vi "Instructor Log.vi"() -> ()   [LabVIEW 2017]
uses:
  <vilib>/OPCUA/controls/Write Status.ctl
  <vilib>/OPCUA/controls/NodeId.ctl
  <vilib>/OPCUA/client/Multiple Write String.vi
  <vilib>/OPCUA/NI OPC UA Client.lvlib
panel:
  out "Log Loop":i32
  out "Send Loop":i32
  out "Chat Window":string
  in  "Node Status":T1 items=["Good"=0, "Uncertain_InitialValue"=1083310080, "Uncertain_LastUsableValue"=1083179008, "Uncertain_SensorNotAccurate"=1083375616, "Uncertain_EngineeringUnitsExceeded"=1083441152, "Bad_NoCommunication"=2150694912, "Bad_NotReadable"=2151284736, "Bad_NotWritable"=2151350272, "Bad_OutOfRange"=2151415808, "Bad_WaitingForInitialData"=2150760448]
  in  "Time Stamp":timestamp
  in  "Enter Text":string
  in  "Node Status":T1 items=["Good"=0, "Uncertain_InitialValue"=1083310080, "Uncertain_LastUsableValue"=1083179008, "Uncertain_SensorNotAccurate"=1083375616, "Uncertain_EngineeringUnitsExceeded"=1083441152, "Bad_NoCommunication"=2150694912, "Bad_NotReadable"=2151284736, "Bad_NotWritable"=2151350272, "Bad_OutOfRange"=2151415808, "Bad_WaitingForInitialData"=2150760448]
  in  "Time Stamp":timestamp
  in  "Stop Chat":bool
  in  "Send":bool
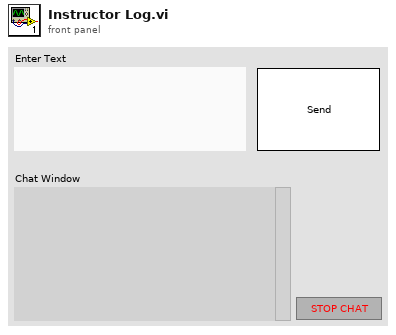
[diagram p1: front panel]
types:
  T1 = typedef "Write Status.ctl" = u32
  T2 = cluster{"message mode":enum16{"None", "Sign", "Sign and Encrypt"}, "security":enum16{"Basic256", "Basic128Rsa15"}}
  T3 = enum16{"open", "replace", "create", "open or create", "replace or create", "replace or create with confirmation"}
  T4 = typedef "OPC UA Client Refnum.ctl" = refnum<k21>
  T5 = typedef "NodeId.ctl" = string
  T6 = cluster{"node ID":T5, "value":string, "timestamp (current time)":timestamp, "node status":T1}
  T7 = cluster{"node ID":T5, "value":string, "timestamp (current time)":timestamp, "node status":T1}[]
  T8 = typedef "Subscription ID.ctl" = u32
  T9 = typedef "Subscription Data Change.ctl" = cluster{"node ID":T5, " value":variant, "timestamp":timestamp, "data type":T10, "status code":T11}
  T10 = typedef "Data Type.ctl" = u16
  T11 = typedef "OPC UA StatusCode.ctl" = u32
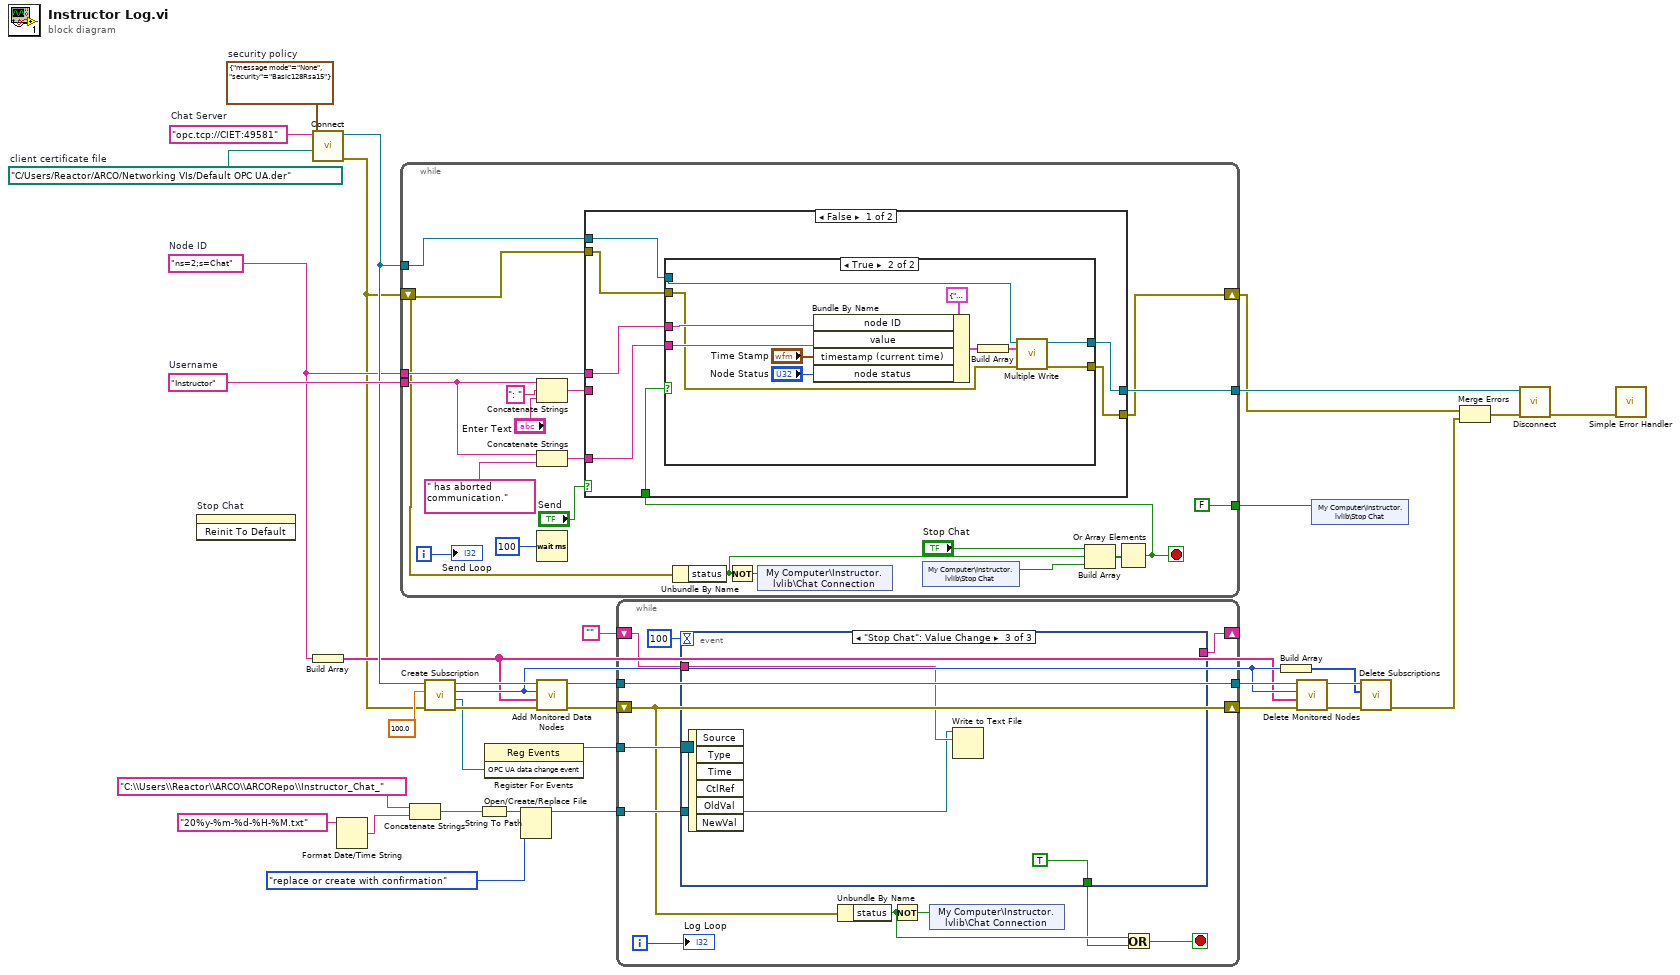
[diagram p0: block diagram]
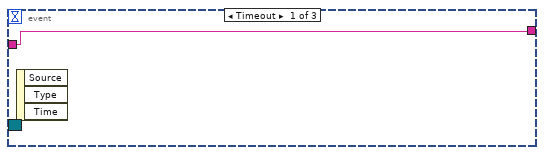
[diagram p2: hidden frame]
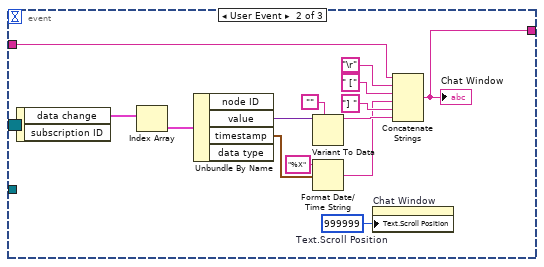
[diagram p3: hidden frame]
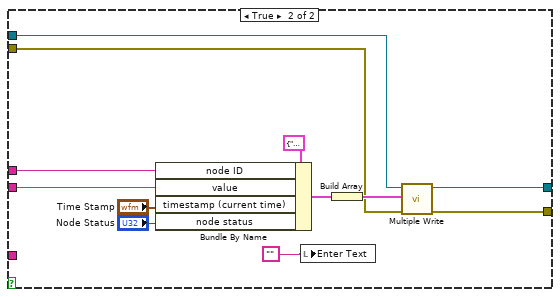
[diagram p5: hidden frame]
diagram:
  w14 = T2 {"message mode"=enum."None", "security"=enum."Basic128Rsa15"}  # security policy
  w15 = path "C:/Users/Reactor/ARCO/Networking VIs/Default OPC UA.der"  # client certificate file
  w19 = "ns=2;s=Chat"  # Node ID
  w33 = "Instructor"  # Username
  w34 = "opc.tcp://CIET:49581"  # Chat Server
  n1 = invoke on="Stop Chat" class="Bool (strict)" method="Reinit To Default"() -> ()  [unwired: 3 in, 3 out]
  n2 = call <vilib>:"Connect.vi"("client certificate file"=w15, "security policy"=w14, "server endpoint URL"=w34) -> ("error out"=w11:errorcluster, "OPC UA client refnum out"=w32:T4)  [unwired: 6 in, 1 out]
  n3 = Build Array(w19) -> (w18:string[])
  n4 = Format Date/Time String(time format string (%c)="20%y-%m-%d-%H-%M.txt") -> (date/time string=w7:string)  [unwired: 2 in]
  n5 = while {
    tunnel: w19 -> [w48]
    tunnel: w33 -> [w53]
    tunnel: w32 -> [w46]
    tunnel: [w47] -> w16
    tunnel: [FALSE] -> w12
    shift-right: [w38] -> w1
    shift-left: w11 -> [w37]
    i -> [w51]
    stop <- w42 stop-if-true
    n6 = Concatenate Strings(w53, ": ", "Enter Text") -> (w49:string)
    n7 = Concatenate Strings(w53, " has aborted communication.") -> (w45:string)
    n8 = Wait (ms)(milliseconds to wait=u32 100) -> ()  [unwired: 1 out]
    n9 = Unbundle By Name(w37) -> ("status"=w41:bool)
    n10 = Not(x=w41) -> (.not. x?=w43:bool)
    n11 = shared-variable "My Computer\\Instructor.lvlib\\Chat Connection"(w43) -> ()  [unwired: 1 in, 1 out]
    n12 = shared-variable "My Computer\\Instructor.lvlib\\Stop Chat"() -> (w36:bool)  [unwired: 1 in, 1 out]
    n13 = Build Array("Stop Chat", w41, w36) -> (w39:bool[])
    n14 = Or Array Elements(Boolean array=w39) -> (logical OR=w42:bool)
    n15 = case shown="False" "Send" {
      tunnel: w49 -> [_ w83]
      tunnel: w48 -> [w61 w82]
      tunnel: [w57 w80] -> w47
      tunnel: [w58 w79] -> w38
      tunnel: w46 -> [w59 w78]
      tunnel: w37 -> [w60 w77]
      tunnel: w42 -> [w63 _]
      tunnel: w45 -> [w62 _]
      frame False {
        n16 = case shown="True" w63 {
          tunnel: w62 -> [_ w71]
          tunnel: w61 -> [_ w70]
          tunnel: w60 -> [w64 w69]
          tunnel: w59 -> [w65 w68]
          tunnel: [w65 w67] -> w57
          tunnel: [w64 w66] -> w58
          frame False {
          }
          frame True {
            n17 = Bundle By Name(cluster=T6 {"node ID"="", "value"="", "timestamp (current time)"=timestamp(0 s since 1904-01-01), "node status"=0} ("request"), "node ID"=w70, "value"=w71, "timestamp (current time)"="Time Stamp", "node status"="Node Status") -> (w74:T6)
            n18 = Build Array(w74) -> (w73:T7)
            n19 = call-poly <vilib>:"Multiple Write.vi"("error in (no error)"=w69, "requests"=w73, "OPC UA client refnum in"=w68) -> ("error out"=w66:errorcluster, "OPC UA client refnum out"=w67:T4)  [unwired: 5 in, 2 out]
          }
        }
      }
      frame True {
        n20 = Bundle By Name(cluster=T6 {"node ID"="", "value"="", "timestamp (current time)"=timestamp(0 s since 1904-01-01), "node status"=0} ("request"), "node ID"=w82, "value"=w83, "timestamp (current time)"="Time Stamp", "node status"="Node Status") -> (w86:T6)
        n21 = local write "Enter Text"("") -> ()
        n22 = Build Array(w86) -> (w85:T7)
        n23 = call-poly <vilib>:"Multiple Write.vi"("error in (no error)"=w77, "requests"=w85, "OPC UA client refnum in"=w78) -> ("error out"=w79:errorcluster, "OPC UA client refnum out"=w80:T4)  [unwired: 5 in, 2 out]
      }
    }
    "Send Loop" <- w51
  }
  n24 = Concatenate Strings("C:\\Users\\Reactor\\ARCO\\ARCORepo\\Instructor_Chat_" ("string"), w7) -> (w5:string)
  n25 = call <vilib>:"Create Subscription.vi"("error in (no error)"=w11, "publishing interval (1000 ms)"=100.0, "OPC UA client refnum in"=w32) -> ("error out"=w30:errorcluster, "OPC UA data change event"=w29:refnum<user-event>, "subscription ID out"=w22:T8, "OPC UA client refnum out"=w31:T4)  [unwired: 4 in, 1 out]
  n26 = String To Path(string=w5) -> (path=w6:path)
  n27 = register-events(w29) -> (reference out=w28:refnum<event-registration>)  [unwired: 2 in, 1 out]
  n28 = Open/Create/Replace File(file path (use dialog)=w6, operation (0:open)=T3."replace or create with confirmation") -> (refnum out=w20:refnum<file>)  [unwired: 4 in, 2 out]
  n29 = call <vilib>:"Add Monitored Data Nodes.vi"("error in (no error)"=w30, "node IDs"=w18, "subscription ID in"=w22, "OPC UA client refnum in"=w31) -> ("error out"=w10:errorcluster, "OPC UA client refnum out"=w26:T4)  [unwired: 4 in, 2 out]
  n30 = while {
    tunnel: w28 -> [w100]
    shift-right: [w98] -> _
    shift-left: "" -> [w99]
    tunnel: w26 -> [w97]
    tunnel: [w97] -> w25
    tunnel: w20 -> [w96]
    shift-right: [w90] -> w9
    shift-left: w10 -> [w90]
    i -> [w95]
    stop <- w92 stop-if-true
    n31 = event shown="[2] \"Stop Chat\": Value Change" {
      selector: w100 -> [_ _ _]
      dyn-events: _ -> [_ _ _]
      timeout: 100 -> [_ _ _]
      tunnel: w99 -> [w101 w104 w118]
      tunnel: [w101 w103 _] -> w98
      tunnel: w96 -> [_ _ w117]
      tunnel: [_ _ TRUE] -> w89
      event Timeout {
        n32 = event-data() -> ()  [unwired: 1 in, 3 out]
      }
      event User Event {
        w102 = u32 999999  # Text.Scroll Position
        n33 = event-data() -> ("data change"=w115:T9[])  [unwired: 1 in, 1 out]
        n34 = Index Array(array=w115) -> (element=w114:T9)  [unwired: 1 in]
        n35 = Unbundle By Name(w114) -> ("value"=w113:variant, "timestamp"=w111:timestamp)  [unwired: 2 out]
        n36 = Variant To Data(type="", Variant=w113) -> (data=w109:string)  [unwired: 1 in, 1 out]
        n37 = Format Date/Time String(time format string (%c)="%X", seconds (now)=w111) -> (date/time string=w107:string)  [unwired: 1 in]
        n38 = property on="Chat Window" class="Str"("Text.Scroll Position"=w102) -> ()  [unwired: 2 in, 2 out]
        n39 = Concatenate Strings(w104, "\r", " [", w107, "] ", w109) -> (w103:string)
        "Chat Window" <- w103
      }
      event "Stop Chat": Value Change {
        n40 = event-data() -> ()  [unwired: 1 in, 6 out]
        n41 = Write to Text File(file (use dialog)=w117, text=w118) -> ()  [unwired: 2 in, 3 out]
      }
    }
    n42 = Unbundle By Name(w90) -> ("status"=w93:bool)
    n43 = Not(x=w93) -> (.not. x?=w91:bool)
    n44 = shared-variable "My Computer\\Instructor.lvlib\\Chat Connection"(w91) -> ()  [unwired: 1 in, 1 out]
    n45 = Or(x=w93, y=w89) -> (x .or. y?=w92:bool)
    "Log Loop" <- w95
  }
  n46 = Build Array(w22) -> (w21:T8[])
  n47 = call <vilib>:"Delete Monitored Nodes.vi"("error in (no error)"=w9, "node IDs"=w18, "subscription ID in"=w22, "OPC UA client refnum in"=w25) -> ("error out"=w23:errorcluster, "OPC UA client refnum out"=w24:T4)  [unwired: 3 in, 3 out]
  n48 = shared-variable "My Computer\\Instructor.lvlib\\Stop Chat"(w12) -> ()  [unwired: 1 in, 1 out]
  n49 = call <vilib>:"Delete Subscriptions.vi"("error in (no error)"=w23, "subscription IDs"=w21, "OPC UA client refnum in"=w24) -> ("error out"=w2:errorcluster)  [unwired: 6 in, 2 out]
  n50 = Merge Errors(w1, w2) -> (w3:errorcluster)
  n51 = call <vilib>:"Disconnect.vi"("error in (no error)"=w3, "OPC UA client refnum in"=w16) -> ("error out"=w35:errorcluster)  [unwired: 9 in]
  n52 = call <vilib>:"Simple Error Handler.vi"("error in (no error)"=w35) -> ()  [unwired: 4 in, 5 out]
